vi "LogHeaders.vi"(8 "error in":errorcluster, 10 "Date and Time":string, 11 "refnum in":refnum<file>) -> (0 "error out":errorcluster, 3 "refnum out":refnum<file>)   [LabVIEW 2017]
uses:
  DataNames.ctl
  <vilib>/Rock Robotics/Network Tables/NT Read Number.vi
  <vilib>/Rock Robotics/Network Tables/NT Read String.vi
panel:
  in  "Headers":T1
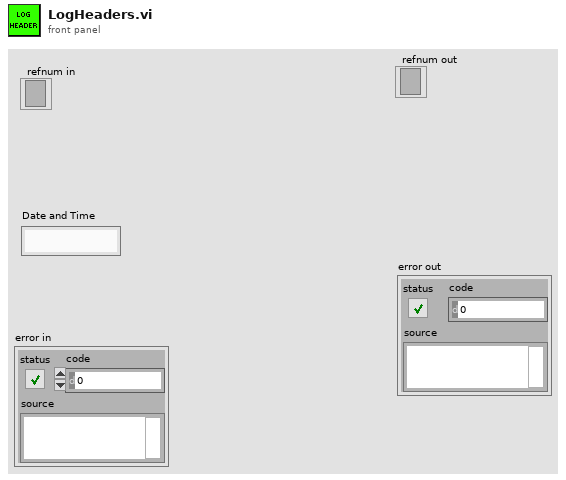
[diagram p1: front panel]
types:
  T1 = typedef "DataNames.ctl" = enum16{"RobotMode", "FMSConnected", "DriveLeft", "DriveRight", "EncoderLeft", "EncoderRight", "Angle", "LocationX", "LocationY", "CPU1", "CPU2", "DriveOperation", "Battery"}
  T2 = typedef "NetComm_MatchType.ctl" = enum32{"None", "Practice", "Qualification", "Elimination"}
  T3 = typedef "WPI_DriverStationPositionInfo.ctl" = enum16{"1", "2", "3"}
  T4 = typedef "WPI_DriverStationAllianceInfo.ctl" = enum16{"Red", "Blue", "Invalid"}
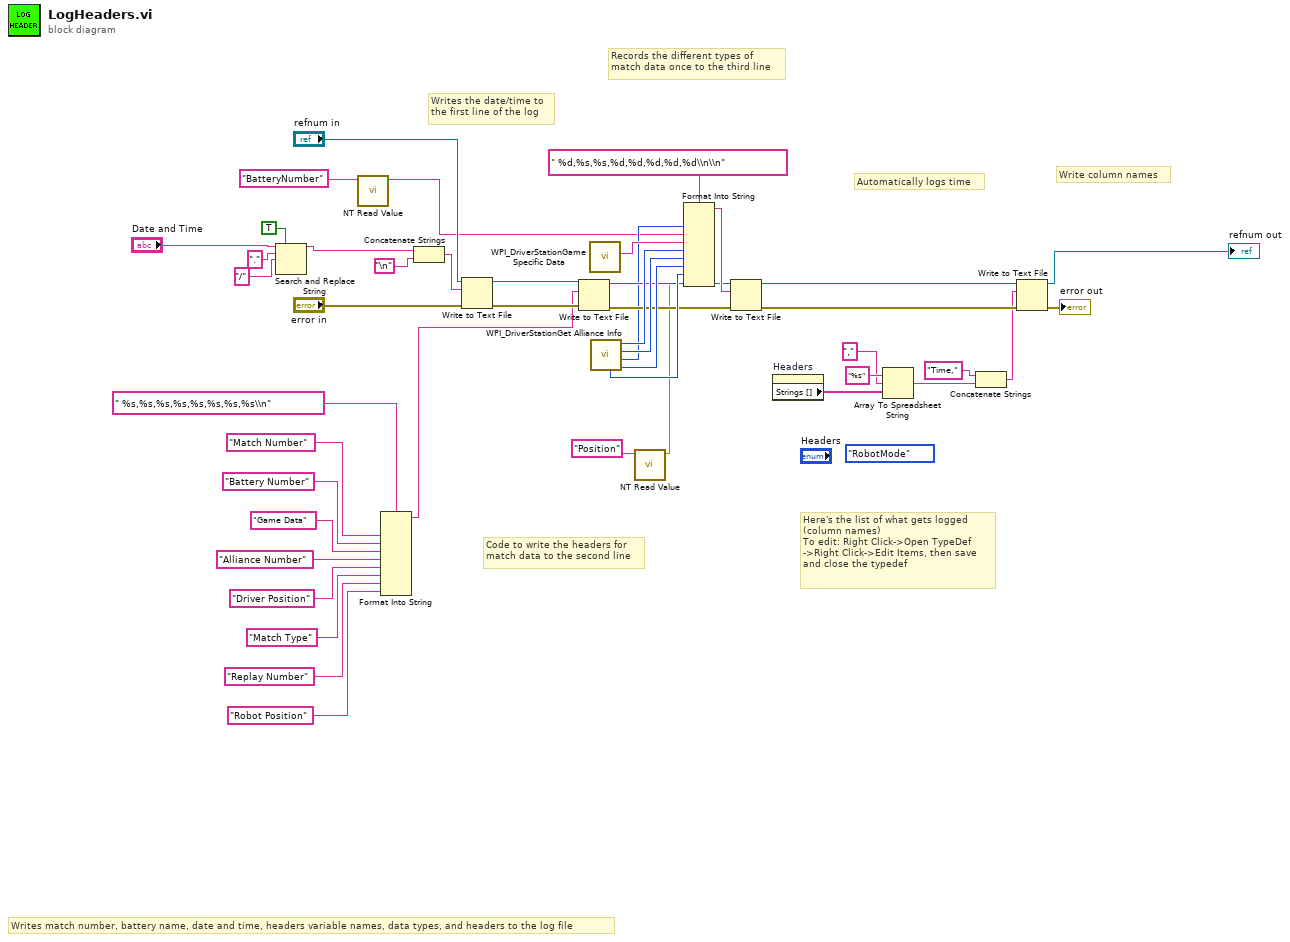
[diagram p0: block diagram]
diagram:
  (unwired) DataNames."RobotMode" ("Name")
  # "Here's the list of what gets logged\n(column names) \nTo edit: Right Click->Open TypeDef\n->Right Click->Edit Items, then save\nand close the typedef"
  # "Automatically logs time"
  # "Write column names"
  # "Records the different types of \nmatch data once to the third line"
  # "Code to write the headers for \nmatch data to the second line"
  # "Writes the date/time to\nthe first line of the log"
  # "Writes match number, battery name, date and time, headers variable names, data types, and headers to the log file"
  n1 = Search and Replace String(replace all?=TRUE ("replace all? (F)"), input string="Date and Time", search string=".", replace string="/" ("search string")) -> (result string=w13:string)  [unwired: 4 in, 3 out]
  n2 = call-poly <vilib>:"NT Read Value.vi"("Name"="BatteryNumber") -> ("String"=w7:string)  [unwired: 9 in, 1 out]
  n3 = Format Into String(format string=" %s,%s,%s,%s,%s,%s,%s,%s\\n", "Match Number" ("input 2"), "Battery Number" ("input 2"), "Game Data" ("input 2"), "Alliance Number" ("input 2"), "Driver Position" ("input 2"), "Match Type" ("input 2"), "Replay Number" ("input 2"), "Robot Position" ("input 2")) -> (resulting string=w18:string)  [unwired: 2 in, 1 out]
  n4 = Concatenate Strings(w13, "\n") -> (w44:string)
  n5 = Write to Text File(file (use dialog)="refnum in", text=w44, error in="error in") -> (refnum out=w30:refnum<file>, error out=w29:errorcluster)  [unwired: 1 in, 1 out]
  n6 = Write to Text File(file (use dialog)=w30, text=w18, error in=w29) -> (refnum out=w27:refnum<file>, error out=w28:errorcluster)  [unwired: 1 in, 1 out]
  n7 = call <vilib>:"WPI_DriverStationGame Specific Data.vi"() -> ("Game Specific Data"=w35:string)  [unwired: 11 in]
  n8 = call <vilib>:"WPI_DriverStationGet Alliance Info.vi"() -> ("Match Type"=w32:T2, "Match Number"=w9:u16, "Position"=w33:T3, "Alliance"=w34:T4, "Replay Number"=w31:u16)  [unwired: 6 in, 1 out]
  n9 = call-poly <vilib>:"NT Read Value.vi"("Name"="Position") -> ("Numeric"=w10:dbl)  [unwired: 9 in, 1 out]
  n10 = Format Into String(format string=" %d,%s,%s,%d,%d,%d,%d,%d\\n\\n", w9, w7, w35, w34, w33, w32, w31, w10) -> (resulting string=w41:string)  [unwired: 2 in, 1 out]
  n11 = Write to Text File(file (use dialog)=w27, text=w41, error in=w28) -> (refnum out=w40:refnum<file>, error out=w39:errorcluster)  [unwired: 1 in, 1 out]
  n12 = property on="Headers" class="Enum (strict)"() -> ("Strings []"=w1:string[])  [unwired: 2 in, 2 out]
  n13 = Array To Spreadsheet String(delimiter (Tab)=",", array=w1, 3:"%s" ("format string")) -> (spreadsheet string=w2:string)
  n14 = Concatenate Strings("Time," ("Column Name"), w2) -> (w5:string)
  n15 = Write to Text File(file (use dialog)=w40, text=w5, error in=w39) -> (refnum out=→"refnum out":refnum<file>, error out=→"error out":errorcluster)  [unwired: 1 in, 1 out]
